vi "Instrumentation Controls.vi"(9 "VISA DS":refnum<visa-resource-name>, 10 "VISA DM":refnum<visa-resource-name>="USB0::0x1AB1::0x0C94::DM3O194400985::INSTR", 11 "VISA DG":refnum<visa-resource-name>="USB0::0x1AB1::0x0641::DG4E202501630::INSTR") -> (1 "DS":bool, 2 "DM":bool, 3 "DG":bool)   [LabVIEW 2018]
doc: "This example shows how to use autosetup and acquire a waveform on a single channel."
uses:
  <instrlib>/RIGOL DS1000 Series/Public/Data/Read (Multiple Waveforms).vi
  <instrlib>/RIGOL DG4000 Series/Public/Configure/Configure Standard Waveform(Square).vi
  <instrlib>/RIGOL DG4000 Series/Public/Configure/Configure Waveform Characteristics(Shape).vi
  <instrlib>/RIGOL DG4000 Series/Public/Configure/Configure Waveform Characteristics(Phase).vi
  <instrlib>/RIGOL DS1000 Series/RIGOL DS1000 Series.lvlib
  <instrlib>/RIGOL DM3058/RIGOL DM3058.lvlib
  <instrlib>/RIGOL DG4000 Series/RIGOL DG4000 Series.lvlib
panel:
  in  "Tab Control":enum32{"DG4062", "DM3068", "DS1204B"}(tab)
  in  "Duty Cycle (50 %) 1":dbl=45.0
  in  "Duty Cycle (50 %) 2":dbl=45.0
  in  "Phase (0 Degree) 2":dbl
  in  "Phase (0 Degree) 1":dbl
  in  "DC Offset (0 V) 1":dbl=1.65
  in  "DC Offset (0 V) 2":dbl=1.65
  in  "Enable Align (F: Disable) 2":bool=TRUE
  in  "Enable Output 2":bool=TRUE
  in  "Enable Align (F: Disable) 1":bool=TRUE
  in  "Enable Output 1":bool=TRUE
  in  "Frequency 1":dbl
  in  "Frequency 2":dbl=180.0
  in  "Waveform Shape (0: Sinusoid) 2":i32(ring)=1 items=["Sinusoid", "Square", "Ramp", "Pulse", "Noise", "User", "Harmonic", "Custom", "DC", "AbsSine", "AbsSineHalf", "AmpALT", "AttALT", "GaussPulse", "NegRamp", "NPulse", "PPulse", "SineTra", "SineVer", "StairDn", "StairUD", "StairUp", "Trapezia", "BandLimited", "Butterworth", "Chebyshev1", "Chebyshev2", "Combin", "CPulse", "CWPulse", "DampedOsc", "DualTone", "Gamma", "GateVibr", "LEMPulse", "MCNoise", "Discharge", "Pahcur", "Quake", "Radar", "Ripple", "RoundHalf", "RoundPM", "StepResp", "SwingOsc", "TV", "Voice", "AM", "FM", "PM", "PWM", "PFM", "Cardiac", "EOG", "EEG", "EMG", "Pulseilogram", "ResSpeed", "LFPulse", "Tens1", "Tens2", "Tens3", "Lgnition", "ISO16750-2 SP", "ISO16750-2 VR", "ISO7637-2 TP1", "ISO7637-2 TP2A", "ISO7637-2 TP2B", "ISO7637-2 TP3A", "ISO7637-2 TP3B", "ISO7637-2 TP4", "ISO7637-2 TP5A", "ISO7637-2 TP5B", "SCR", "Surge", "Airy", "Besselj", "Bessely", "Cauchy", "Cubic", "Dirichlet", "Erf", "Erfc", "Erfclnv", "Erflnv", "ExpFall", "ExpRise", "Gauss", "HaverSine", "Laguerre", "Laplace", "Legend", "Log", "LogNormal", "Lorentz", "Maxwell", "Rayleigh", "Versiera", "Weibull", "ARB_X2", "CosH", "CosInt", "Cot", "CotHCon", "CotHPro", "CscCon", "CscPro", "CscHCon", "CscHPro", "RecipCon", "RecipPro", "SecCon", "SecPro", "SecH", "Sinc", "SinH", "SinInt", "Sqrt", "Tan", "TanH", "ACos", "ACosH", "ACotCon", "ACotPro", "ACotHCon", "ACotHPro", "ACscCon", "ACscPro", "ACscHCon", "ACscHPro", "ASecCon", "ASsePro", "ASecH", "ASin", "ASinH", "ATan", "ATanH", "Barlett", "BarthannWin", "Blackman", "BlackmanH", "BlackmanWin", "Boxcar", "ChebWin", "FlattopWin", "Hamming", "Hanning", "Kaiser", "NuttallWin", "ParzenWin", "TaylorWin", "Triang", "TukeyWin"]
  in  "Output Channel (1: Channel 1) 2":i32(ring)=2 items=["Channel 1"=1, "Channel 2"=2]
  in  "Amplitude (0.1 Vpp) 2":dbl=3.3
  in  "Waveform Shape (0: Sinusoid) 1":i32(ring)=1 items=["Sinusoid", "Square", "Ramp", "Pulse", "Noise", "User", "Harmonic", "Custom", "DC", "AbsSine", "AbsSineHalf", "AmpALT", "AttALT", "GaussPulse", "NegRamp", "NPulse", "PPulse", "SineTra", "SineVer", "StairDn", "StairUD", "StairUp", "Trapezia", "BandLimited", "Butterworth", "Chebyshev1", "Chebyshev2", "Combin", "CPulse", "CWPulse", "DampedOsc", "DualTone", "Gamma", "GateVibr", "LEMPulse", "MCNoise", "Discharge", "Pahcur", "Quake", "Radar", "Ripple", "RoundHalf", "RoundPM", "StepResp", "SwingOsc", "TV", "Voice", "AM", "FM", "PM", "PWM", "PFM", "Cardiac", "EOG", "EEG", "EMG", "Pulseilogram", "ResSpeed", "LFPulse", "Tens1", "Tens2", "Tens3", "Lgnition", "ISO16750-2 SP", "ISO16750-2 VR", "ISO7637-2 TP1", "ISO7637-2 TP2A", "ISO7637-2 TP2B", "ISO7637-2 TP3A", "ISO7637-2 TP3B", "ISO7637-2 TP4", "ISO7637-2 TP5A", "ISO7637-2 TP5B", "SCR", "Surge", "Airy", "Besselj", "Bessely", "Cauchy", "Cubic", "Dirichlet", "Erf", "Erfc", "Erfclnv", "Erflnv", "ExpFall", "ExpRise", "Gauss", "HaverSine", "Laguerre", "Laplace", "Legend", "Log", "LogNormal", "Lorentz", "Maxwell", "Rayleigh", "Versiera", "Weibull", "ARB_X2", "CosH", "CosInt", "Cot", "CotHCon", "CotHPro", "CscCon", "CscPro", "CscHCon", "CscHPro", "RecipCon", "RecipPro", "SecCon", "SecPro", "SecH", "Sinc", "SinH", "SinInt", "Sqrt", "Tan", "TanH", "ACos", "ACosH", "ACotCon", "ACotPro", "ACotHCon", "ACotHPro", "ACscCon", "ACscPro", "ACscHCon", "ACscHPro", "ASecCon", "ASsePro", "ASecH", "ASin", "ASinH", "ATan", "ATanH", "Barlett", "BarthannWin", "Blackman", "BlackmanH", "BlackmanWin", "Boxcar", "ChebWin", "FlattopWin", "Hamming", "Hanning", "Kaiser", "NuttallWin", "ParzenWin", "TaylorWin", "Triang", "TukeyWin"]
  in  "Output Channel (1: Channel 1)":i32(ring)=1 items=["Channel 1"=1, "Channel 2"=2]
  in  "Amplitude (0.1 Vpp) 1":dbl=3.3
  out "Measurement 3":dbl(knob) scale=0.0..5.0
  in  "Function (0: DC Volts) 2":u16(ring) items=["DC Volts", "AC Volts", "DC Current", "AC Current", "2-Wire Resistance", "4-Wire Resistance"]
  in  "Manual Range (1.0) 2":dbl=1.0
  in  "Auto Range (T: Enable) 2":bool=TRUE
  out "Measurement 4":dbl
  in  "Absolute Resolution (0: 5.5 Rate:Slow)":u16(ring) items=["5.5 Rate:Slow", "4.5 Rate:Middle", "4.5 Rate:Fast", "3.5 Rate", "6.5 Rate"]
  out "Waveform Data":waveform(dbl)[](graph)
  in  "Timeout (10000 ms)":u32=10000
  in  "Stop":bool
  in  "Channel (0: Channel 1)":u16[](array[ring]) items=["Channel 1", "Channel 2", "Channel 3", "Channel 4"]
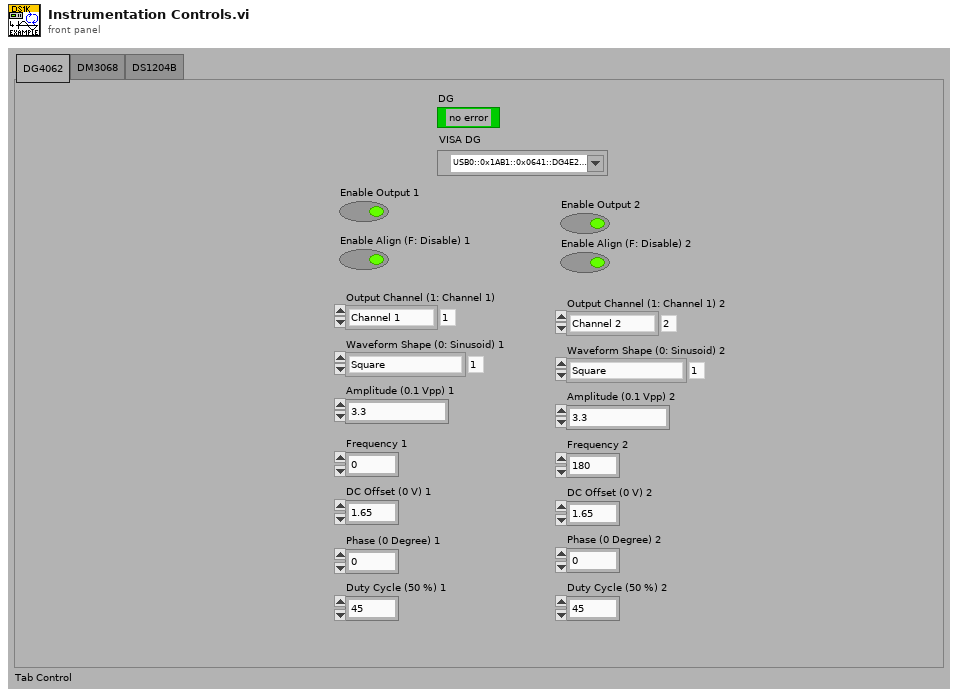
[diagram p1: front panel]
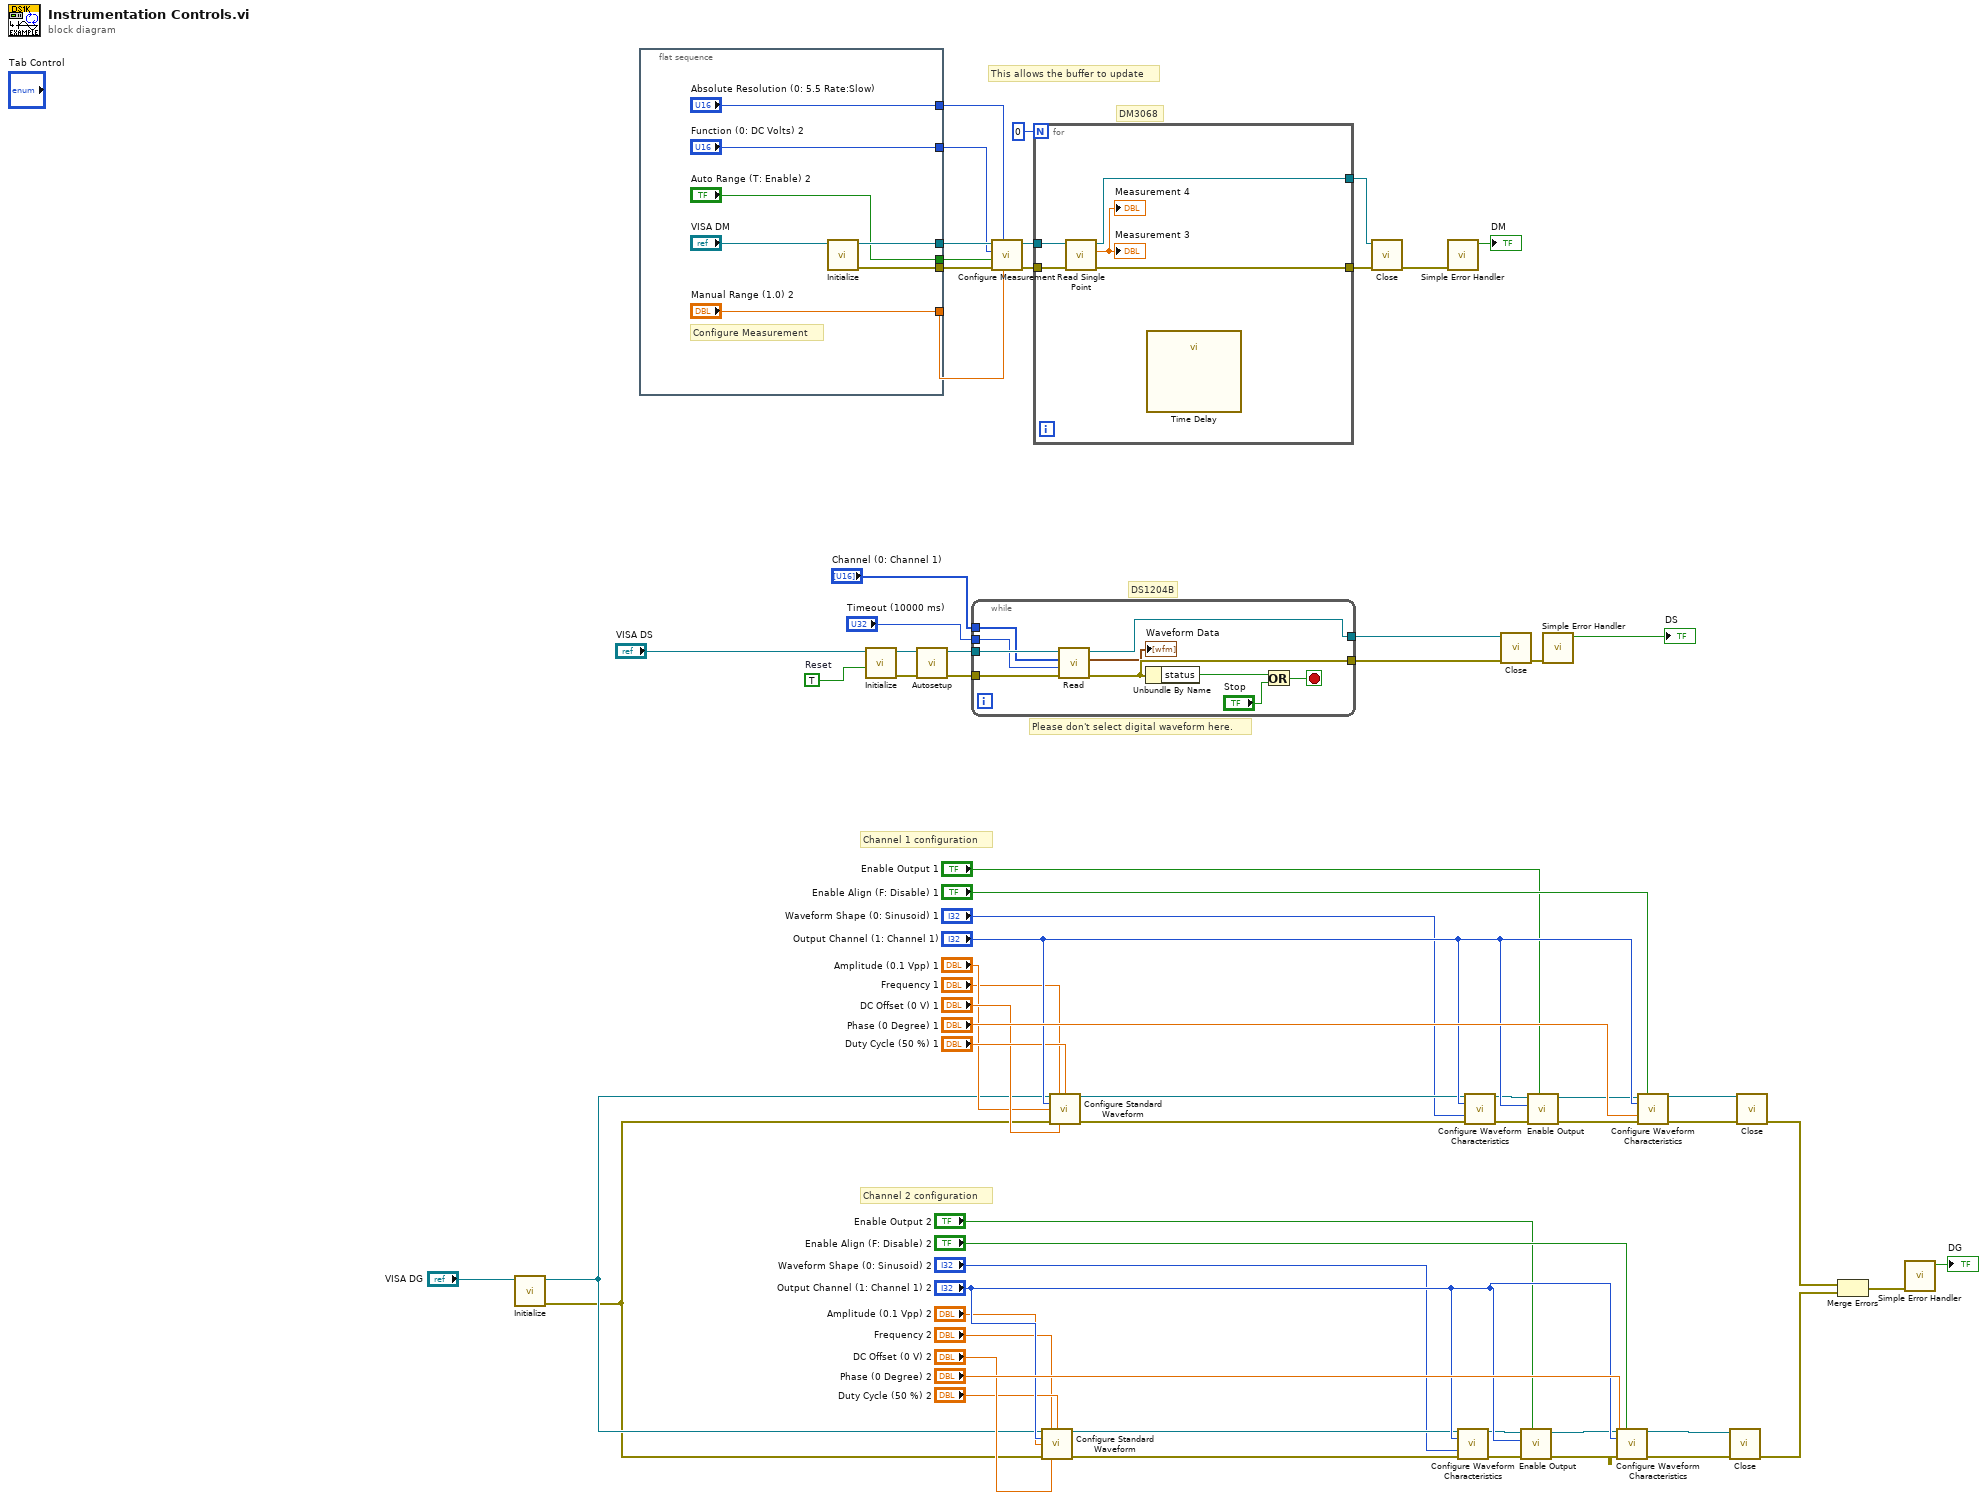
[diagram p0: block diagram]
diagram:
  w52 = TRUE  # Reset
  # "Channel 2 configuration"
  # "Channel 1 configuration"
  # "DS1204B"
  # "This allows the buffer to update"
  # "DM3068"
  # "Please don't select digital waveform here."
  n1 = call <instrlib>:"Initialize.vi"("VISA resource name"="VISA DG") -> ("error out"=w11:errorcluster, "VISA resource name out"=w13:refnum<visa-resource-name>)  [unwired: 4 in, 5 out]
  n2 = flat-sequence {
    tunnel: [w72] -> w57
    tunnel: [w71] -> w56
    tunnel: ["Function (0: DC Volts) 2"] -> w55
    tunnel: ["Manual Range (1.0) 2"] -> w54
    tunnel: ["Auto Range (T: Enable) 2"] -> w53
    tunnel: ["Absolute Resolution (0: 5.5 Rate:Slow)"] -> w2
    frame #0 {
      # "Configure Measurement"
      n3 = call <instrlib>:"Initialize.vi"("VISA resource name"="VISA DM") -> ("error out"=w71:errorcluster, "VISA resource name out"=w72:refnum<visa-resource-name>)  [unwired: 4 in, 5 out]
    }
  }
  n4 = call <instrlib>:"Initialize.vi"("Reset (True)"=w52, "VISA resource name"="VISA DS") -> ("error out"=w59:errorcluster, "VISA resource name out"=w58:refnum<visa-resource-name>)  [unwired: 2 in, 6 out]
  n5 = call <instrlib>:"Autosetup.vi"("error in (no error)"=w59, "VISA resource name"=w58) -> ("error out"=w51:errorcluster, "VISA resource name out"=w50:refnum<visa-resource-name>)  [unwired: 8 out]
  n6 = while {
    tunnel: w50 -> [w83]
    tunnel: w51 -> [w82]
    tunnel: [w81] -> w65
    tunnel: [w79] -> w64
    tunnel: "Channel (0: Channel 1)" -> [w75]
    tunnel: "Timeout (10000 ms)" -> [w74]
    stop <- w80 stop-if-true
    n7 = call-poly <instrlib>:"Read.vi"("error in (no error)"=w82, "Timeout (10000 ms)"=w74, "Channels"=w75, "VISA resource name"=w83) -> ("error out"=w79:errorcluster, "Waveform Data"=→"Waveform Data":waveform(dbl)[], "VISA resource name out"=w81:refnum<visa-resource-name>)  [unwired: 5 out]
    n8 = Unbundle By Name(w79) -> ("status"=w78:bool)
    n9 = Or(x=w78, y="Stop") -> (x .or. y?=w80:bool)
  }
  n10 = call <instrlib>:"Configure Measurement.vi"("Manual Range (1.00)"=w54, "Absolute Resolution (0: 5.5 Rate:Slow)"=w2, "error in (no error)"=w56, "Auto Range (T:Enable)"=w53, "Function (0: DC Volts)"=w55, "VISA resource name"=w57) -> ("error out"=w49:errorcluster, "VISA resource name out"=w48:refnum<visa-resource-name>)  [unwired: 4 out]
  n11 = for {
    N: 0 -> [_]
    tunnel: w48 -> [w88]
    tunnel: [w86] -> w62
    tunnel: w49 -> [w87]
    tunnel: [w85] -> w61
    n12 = call <instrlib>:"Read Single Point.vi"("error in (no error)"=w87, "VISA resource name"=w88) -> ("error out"=w85:errorcluster, "Measurement"=→"Measurement 3" →"Measurement 4":dbl, "VISA resource name out"=w86:refnum<visa-resource-name>)  [unwired: 7 out]
    n13 = call "Time Delay"() -> ()  [unwired: 11 in, 1 out]
  }
  n14 = call-poly <instrlib>:"Configure Standard Waveform.vi"("VISA resource name"=w13, "Frequency (1000 Hz)"="Frequency 2", "Output Channel (1: Channel 1)"="Output Channel (1: Channel 1) 2", "Amplitude (5 Vpp)"="Amplitude (0.1 Vpp) 2", "error in (no error)"=w11, "Offset (0)"="DC Offset (0 V) 2", "Duty Cycle (50 %)"="Duty Cycle (50 %) 2") -> ("VISA resource name out"=w18:refnum<visa-resource-name>, "error out"=w19:errorcluster)  [unwired: 7 in]
  n15 = call-poly <instrlib>:"Configure Standard Waveform.vi"("VISA resource name"=w13, "Frequency (1000 Hz)"="Frequency 1", "Output Channel (1: Channel 1)"="Output Channel (1: Channel 1)", "Amplitude (5 Vpp)"="Amplitude (0.1 Vpp) 1", "error in (no error)"=w11, "Offset (0)"="DC Offset (0 V) 1", "Duty Cycle (50 %)"="Duty Cycle (50 %) 1") -> ("VISA resource name out"=w20:refnum<visa-resource-name>, "error out"=w21:errorcluster)  [unwired: 7 in]
  n16 = call <instrlib>:"Close.vi"("error in (no error)"=w61, "VISA resource name"=w62) -> ("error out"=w63:errorcluster)  [unwired: 9 out]
  n17 = call <vilib>:"Simple Error Handler.vi"("error in (no error)"=w63) -> ("error?"=→"DM":bool)  [unwired: 1 in, 7 out]
  n18 = call-poly <instrlib>:"Configure Waveform Characteristics.vi"("VISA resource name"=w18, "Output Channel (1: Channel 1)"="Output Channel (1: Channel 1) 2", "Waveform Shape (0: Sinusoid)"="Waveform Shape (0: Sinusoid) 2", "error in (no error)"=w19) -> ("VISA resource name out"=w14:refnum<visa-resource-name>, "error out"=w15:errorcluster)  [unwired: 10 out]
  n19 = call-poly <instrlib>:"Configure Waveform Characteristics.vi"("VISA resource name"=w20, "Output Channel (1: Channel 1)"="Output Channel (1: Channel 1)", "Waveform Shape (0: Sinusoid)"="Waveform Shape (0: Sinusoid) 1", "error in (no error)"=w21) -> ("VISA resource name out"=w16:refnum<visa-resource-name>, "error out"=w17:errorcluster)  [unwired: 10 out]
  n20 = call <instrlib>:"Close.vi"("error in (no error)"=w64, "VISA resource name"=w65) -> ("error out"=w66:errorcluster)  [unwired: 9 out]
  n21 = call <instrlib>:"Enable Output.vi"("Enable Output (T: Enable)"="Enable Output 2", "error in (no error)"=w15, "Output Channel (1: Channel 1)"="Output Channel (1: Channel 1) 2", "VISA resource name"=w14) -> ("error out"=w36:errorcluster, "VISA resource name out"=w39:refnum<visa-resource-name>)  [unwired: 6 out]
  n22 = call <instrlib>:"Enable Output.vi"("Enable Output (T: Enable)"="Enable Output 1", "error in (no error)"=w17, "Output Channel (1: Channel 1)"="Output Channel (1: Channel 1)", "VISA resource name"=w16) -> ("error out"=w33:errorcluster, "VISA resource name out"=w30:refnum<visa-resource-name>)  [unwired: 6 out]
  n23 = call <vilib>:"Simple Error Handler.vi"("error in (no error)"=w66) -> ("error?"=→"DS":bool)  [unwired: 1 in, 7 out]
  n24 = call-poly <instrlib>:"Configure Waveform Characteristics.vi"("VISA resource name"=w39, "Enable Align (F: Disable)"="Enable Align (F: Disable) 2", "Output Channel (1: Channel 1)"="Output Channel (1: Channel 1) 2", "Phase (0 Degree)"="Phase (0 Degree) 2", "error in (no error)"=w36) -> ("VISA resource name out"=w35:refnum<visa-resource-name>, "error out"=w37:errorcluster)  [unwired: 9 in]
  n25 = call-poly <instrlib>:"Configure Waveform Characteristics.vi"("VISA resource name"=w30, "Enable Align (F: Disable)"="Enable Align (F: Disable) 1", "Output Channel (1: Channel 1)"="Output Channel (1: Channel 1)", "Phase (0 Degree)"="Phase (0 Degree) 1", "error in (no error)"=w33) -> ("VISA resource name out"=w31:refnum<visa-resource-name>, "error out"=w32:errorcluster)  [unwired: 9 in]
  n26 = call <instrlib>:"Close.vi"("error in (no error)"=w37, "VISA resource name"=w35) -> ("error out"=w10:errorcluster)  [unwired: 9 out]
  n27 = call <instrlib>:"Close.vi"("error in (no error)"=w32, "VISA resource name"=w31) -> ("error out"=w9:errorcluster)  [unwired: 9 out]
  n28 = Merge Errors(w9, w10) -> (w3:errorcluster)
  n29 = call <vilib>:"Simple Error Handler.vi"("error in (no error)"=w3) -> ("error?"=→"DG":bool)  [unwired: 1 in, 7 out]
